vi "2100_SP3T_SMU_Meas and Calculate Resitance_No Publish Data_Rfree.vi"(0 "Semiconductor Module Context":T1, 1 "Current  Level":dbl=-0.01, 5 "Pins":string[](array[string]), 11 "error in (no error)":errorcluster) -> (4 "Semiconductor Module Context Out":T1, 6 "Mean_Meas_Current":dbl[](array[numeric]), 10 "Individual_R_Meas":dbl[](array[numeric]), 13 "Meas_Current_RF3":dbl[](array[numeric]), 14 "Mean_Meas_Voltage":dbl[](array[numeric]), 15 "error Out":errorcluster)   [LabVIEW 2013]
uses:
  <vilib>/NI_TestStand_SemiconductorModule/NI_TestStand_Semiconductor_Module.lvlibp/PinMap/General/SemiconductorModuleContext.ctl
  <vilib>/NI_TestStand_SemiconductorModule/NI_TestStand_Semiconductor_Module.lvlibp/PinMap/DC Power/PinsToNIDCPowerSessions.vi
  <vilib>/NI_TestStand_SemiconductorModule/NI_TestStand_Semiconductor_Module.lvlibp
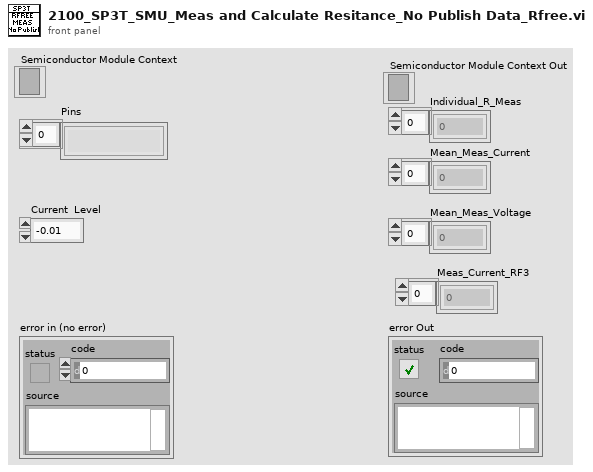
[diagram p1: front panel]
types:
  T1 = typedef "NI_TestStand_Semiconductor_Module.lvlibp/SemiconductorModuleContext.ctl" = refnum<k7>
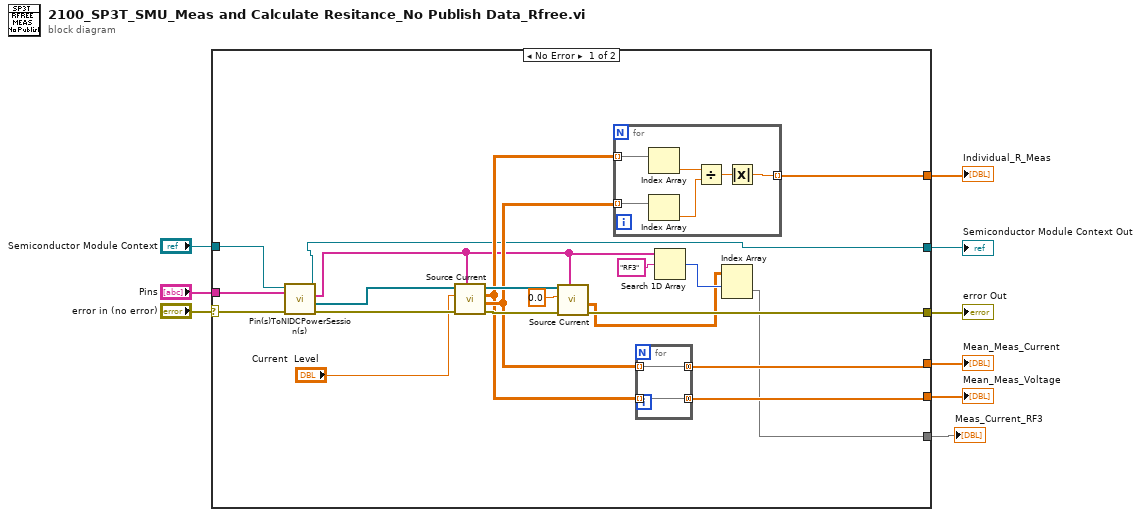
[diagram p0: block diagram]
diagram:
  n1 = case shown="No Error" "error in (no error)" {
    selector: "error in (no error)" -> [w30 w40]
    tunnel: "Semiconductor Module Context" -> [w28 w39]
    tunnel: "Pins" -> [w29 _]
    tunnel: [w16 w40] -> w6
    tunnel: [w15 w39] -> w5
    tunnel: [w25 _] -> w4
    tunnel: [w20 _] -> w3
    tunnel: [w18 _] -> w2
    tunnel: [w10 _] -> w1
    frame No Error {
      n2 = call-poly <vilib>:"Pin(s)ToNIDCPowerSession(s).vi"("error in (no error)"=w30, "Pins"=w29, "Semiconductor Module Context"=w28) -> ("error out"=w27:errorcluster, "Instrument Sessions"=w26:refnum<k15>[], "Channel Lists"=w14:string[], "Semiconductor Module Context Out"=w15:T1)  [unwired: 4 in, 1 out]
      n3 = call "Source Current.vi"("Channel Lists"=w14, "error in (no error)"=w27, "current level"="Current  Level", "Instrument Sessions In"=w26) -> ("error out"=w23:errorcluster, "current measurements"=w21:dbl[][], "voltage measurements"=w19:dbl[][], "Instrument Sessions Out"=w22:refnum<k15>[])  [unwired: 4 in]
      n4 = call "Source Current.vi"("Channel Lists"=w14, "error in (no error)"=w23, "current level"=0.0, "Instrument Sessions In"=w22) -> ("error out"=w16:errorcluster, "current measurements"=w11:dbl[][])  [unwired: 4 in, 2 out]
      n5 = for {
        tunnel: [w37] -> w25 mode=indexing
        tunnel: w21 -> [w36] mode=indexing
        tunnel: w19 -> [w35] mode=indexing
        n6 = Index Array(array=w35) -> (element=w34:dbl)  [unwired: 1 in]
        n7 = Index Array(array=w36) -> (element=w33:dbl)  [unwired: 1 in]
        n8 = Divide(x=w34, y=w33) -> (x/y=w38:dbl)
        n9 = Absolute Value(x=w38) -> (abs(x)=w37:dbl)
      }
      n10 = for {
        tunnel: w21 -> [w32] mode=indexing
        tunnel: [w32] -> w20 mode=concatenating
        tunnel: w19 -> [w31] mode=indexing
        tunnel: [w31] -> w18 mode=concatenating
      }
      n11 = Search 1D Array(1D array=w14, element="RF3") -> (index of element=w12:i32)  [unwired: 1 in]
      n12 = Index Array(array=w11, index (row)=w12) -> (element=w10:dbl[])  [unwired: 1 in]
    }
    frame Error {
    }
  }
  "error Out" <- w6
  "Semiconductor Module Context Out" <- w5
  "Individual_R_Meas" <- w4
  "Mean_Meas_Current" <- w3
  "Mean_Meas_Voltage" <- w2
  "Meas_Current_RF3" <- w1
